vi "Execute Sequence.vi"(4 "Sequence Progress":refnum<vi>, 6 "Pulse Sequence Type":T1, 7 "Sum?":bool=TRUE, 8 "error in (no error)":errorcluster, 9 "file path (use dialog)":path, 10 "Save File":bool, 11 "class objects in":T2) -> (0 "error out":errorcluster, 1 "Stop?":bool, 2 "CMD STR Array":string[](array[string]), 3 "class objects out":T2)   [LabVIEW 2011]
uses:
  Controls/Class Objects.ctl
  Modules/File/Configuration/Configuration.lvclass
  Modules/Hardware/Power Supply/Power Supply.lvclass
  Modules/Hardware/NMR/NMR.lvclass
  Modules/File/TDMS/TDMS.lvclass
  Controls/NMR Pulse Sequence Type.ctl
  Controls/User Interface Action.ctl
  Controls/TDMS File Handling.ctl
  Functional Globals/Pulse Parameters.ctl
  <vilib>/Utility/file.llb/Write To Spreadsheet File (I64).vi
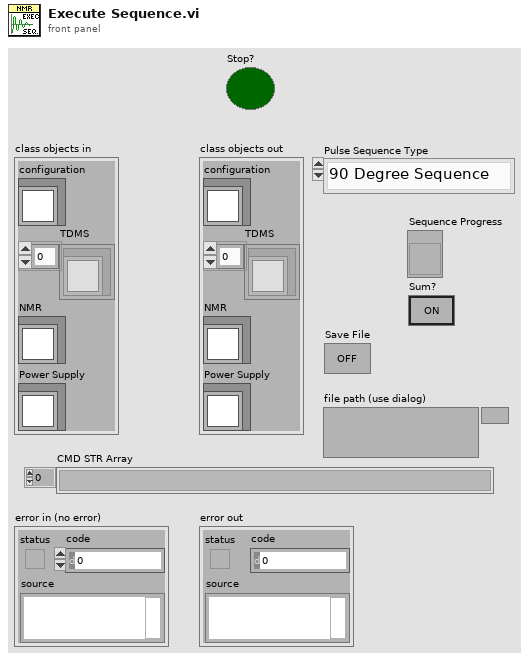
[diagram p1: front panel]
types:
  T1 = typedef "NMR Pulse Sequence Type.ctl" = enum16{"90 Degree Sequence", "CPMG Pulse Sequence", "T1 Pulse Sequence"}
  T2 = typedef "Class Objects.ctl" = cluster{"configuration":refnum<class "Configuration.lvclass">, "TDMS":refnum<class "TDMS.lvclass">[], "Power Supply":refnum<class "Power Supply.lvclass">, "NMR":refnum<class "NMR.lvclass">}
  T3 = typedef "User Interface Action.ctl" = enum16{"Initialize", "Update Real Channel", "Update Imag Channel", "Update Re/Im channel @ Hardware Ctrl", "Pulse Sequence", "Visibility Front Panel Controls", "Report Custom Errors", "Set Pulse Sequence Type", "Update Pulse Timings", "Update Transfer Time", "Update Status Bar", "Set Sequence Progress", "Set 90 Degree Pulse Sequence Params", "Set CMPG Pulse Sequence Parms", "Set T1 Pulse Sequence Params", "Stop"}
  T4 = typedef "TDMS File Handling.ctl" = enum16{"Add TDMS File", "Get Active TDMS File", "Set Active TDMS File", "Set Active TDMS File Index"}
  T5 = typedef "Pulse Parameters.ctl" = enum16{"Initialize", "Set T1 Pulse Settings", "Set 90 Degree Pulse Settings", "Set CPMG Pulse Settings", "Get T1 Settings", "Get CPMG Settings", "Get 90 Degree Settings"}
  T6 = typedef "90D_Delay Settings.ctl" = cluster{"Delay d1":dbl, "Delay d2":dbl, "d1 Unit":u8, "d2 Unit":u8}
  T7 = typedef "90D_Preliminary Settings.ctl" = cluster{"Nº of Scans (ns)":u16, "Pulse Frequency":dbl}
  T8 = typedef "90D_Pulse Settings.ctl" = cluster{"Duration Signal P1":dbl, "Power Level":u16, "Phase":u16, "P1 Units":u8}
  T9 = typedef "Acquisition Settings.ctl" = cluster{"Number Samples":u16, "Time Between Points":dbl, "Unit":u8}
  T10 = cluster{"Delay Settings":T6, "Preliminary Settings":T7, "Pulse Settings":T8, "Acquisition Settings":T9}
  T11 = cluster{"D1 Real Time":ext, "D2 Real Time":ext, "P1 Real Time":ext, "AQS Real Time":ext}
  T12 = typedef "CPMG_Delay Settings.ctl" = cluster{"Delay d1":dbl, "Delay d2":dbl, "d1 Unit":u8, "d2 Unit":u8, "Delay d3":dbl, "d3 Unit":u8, "Delay d4":dbl, "d4 Unit":u8}
  T13 = typedef "CPMG_Preliminary Settings.ctl" = cluster{"Nº of Scans (ns)":u16, "Pulse Frequency":dbl, "Nº of Echoes (ne)":u16}
  T14 = typedef "CPMG_Pulse Settings.ctl" = cluster{"Duration Signal P1":dbl, "Power Level P1":u16, "Phase P1":u16, "P1 Unit":u8, "Duration Signal P2":dbl, "Power Level P2":u16, "Phase P2":u16, "P2 Unit":u8}
  T15 = cluster{"Acquisition Settings":T9, "Delay Settings":T12, "Preliminary Settings":T13, "Pulse Settings":T14}
  T16 = cluster{"Real Time d4":ext, "Real Time d3":ext, "Real Time P2":ext, "Real Time d2":ext, "Real Time P1":ext, "Real Time d1":ext, "Real Time AQS":ext}
  T17 = typedef "T1_Preliminary Settings.ctl" = cluster{"Nº of Scans (ns)":u16, "Pulse Frequency":dbl, "Nº of Vd":u16}
  T18 = typedef "T1_Pulse Settings.ctl" = cluster{"Duration Signal P2":dbl, "Power Level P2":u16, "Phase P2":u16, "P2 Unit":u8, "Duration Signal P1":dbl, "Power Level P1":u16, "Phase P1":u16, "P1 Unit":u8}
  T19 = typedef "T1_Delay Settings.ctl" = cluster{"Delay d1":dbl, "Delay d2":dbl, "d1 Unit":u8, "d2 Unit":u8, "Delay d30":dbl, "d30 Unit":u8, "Vd Unit":u8, "Vd Values":string}
  T20 = cluster{"Preliminary Settings":T17, "Pulse Settings":T18, "Acquisition Settings":T9, "Delay Settings":T19}
  T21 = cluster{"Real Time P1":ext, "Real Time P2":ext, "Real Time d1":ext, "Real Time d2":ext, "Real Time d30":ext, "Real Time AQS":ext}
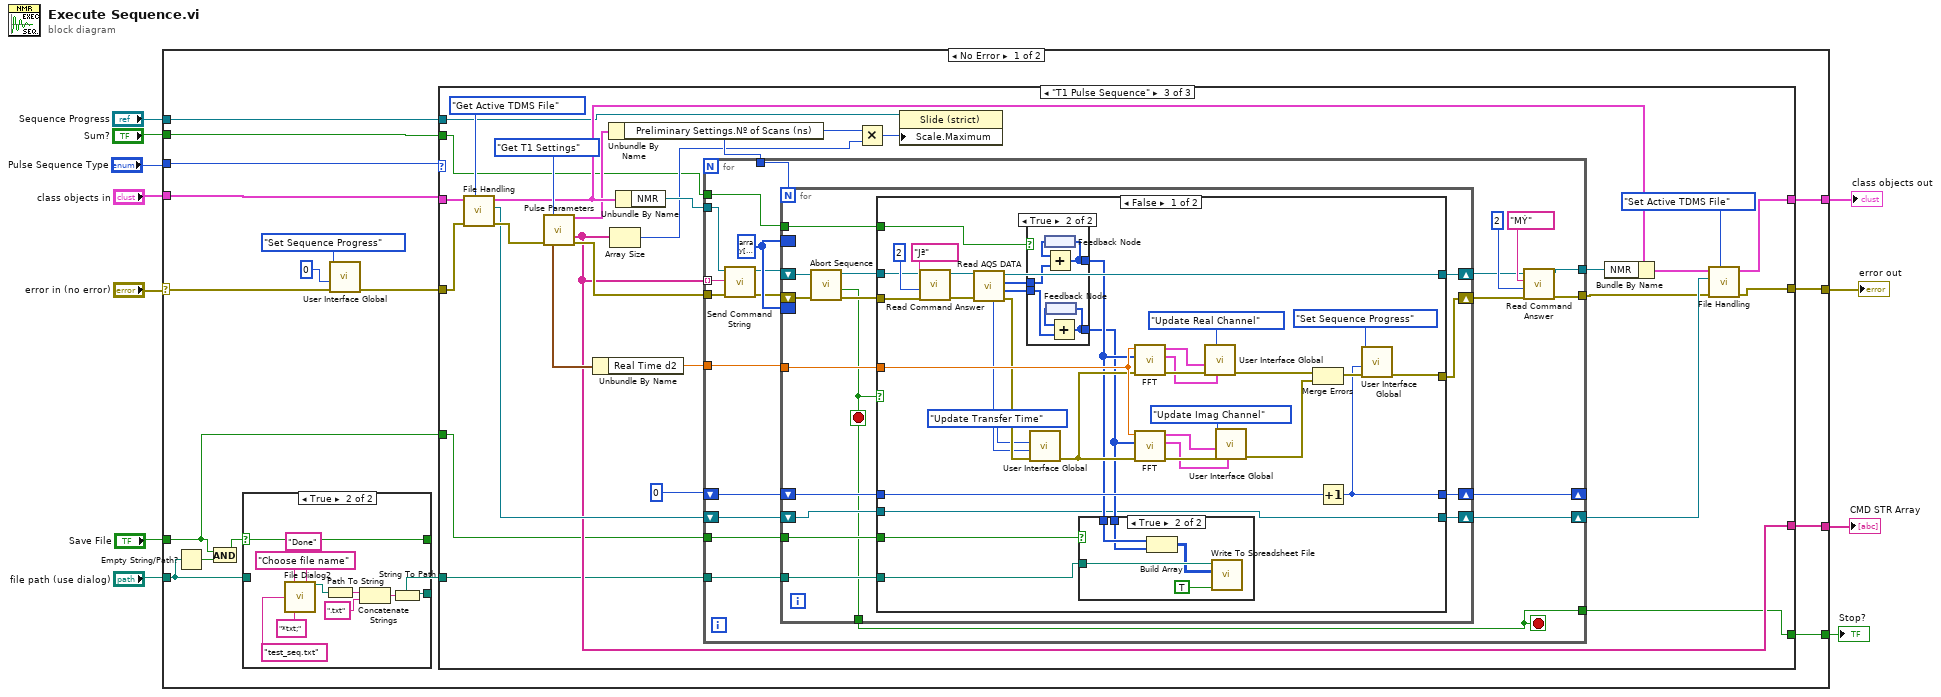
[diagram p0: block diagram]
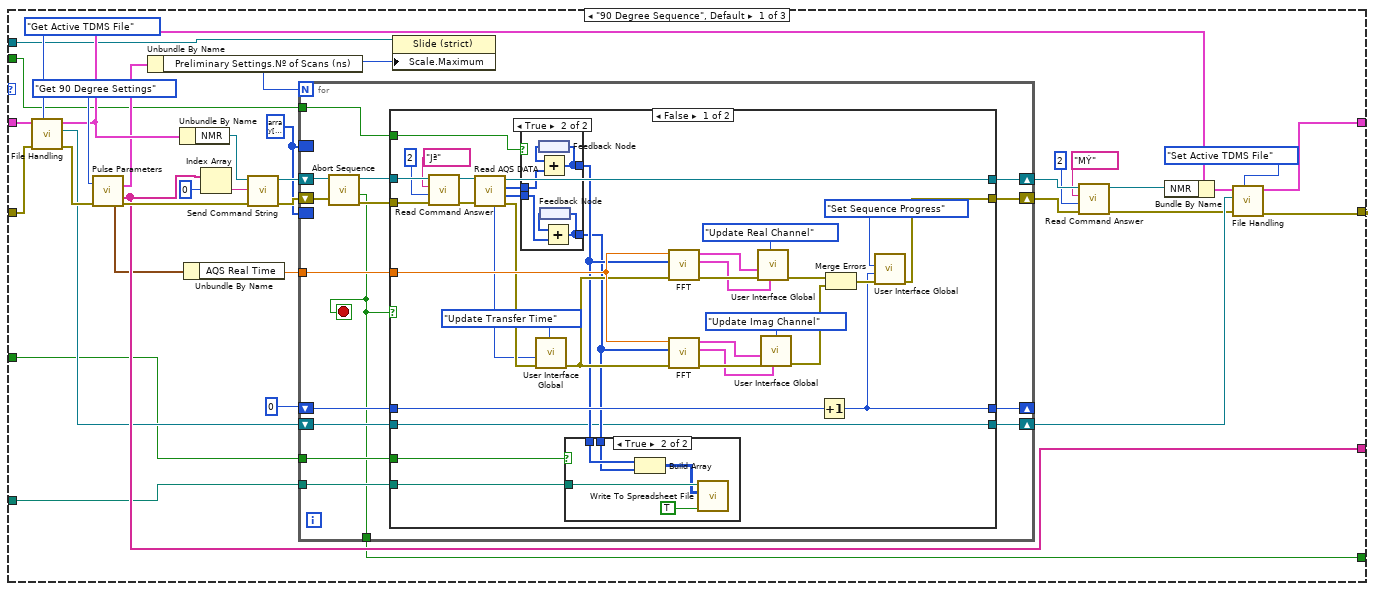
[diagram p3: hidden frame]
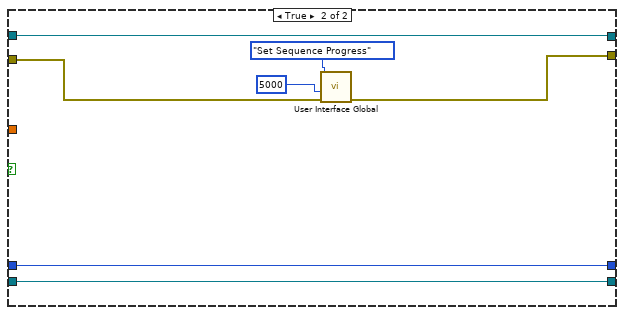
[diagram p6: hidden frame]
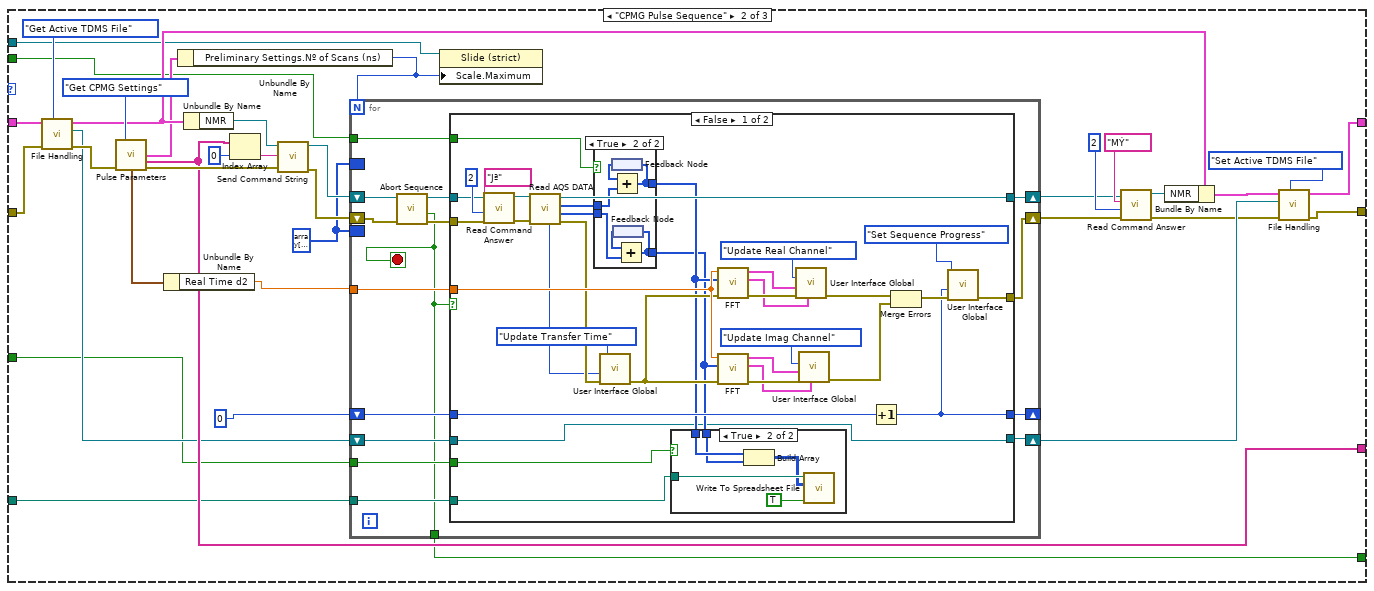
[diagram p7: hidden frame]
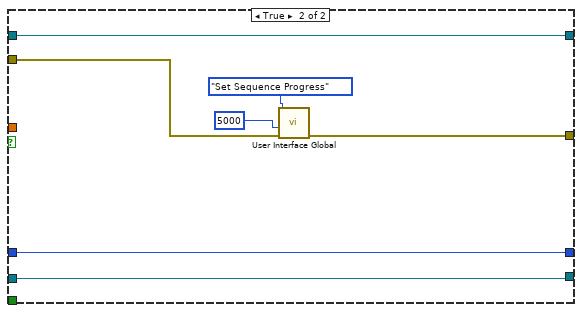
[diagram p10: hidden frame]
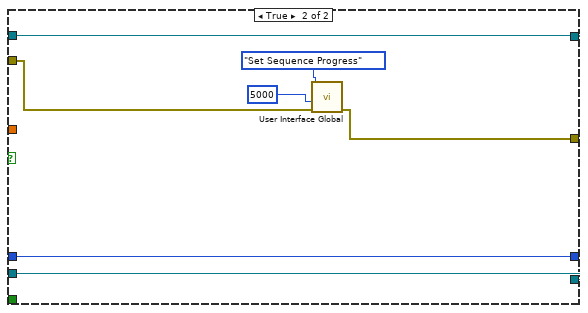
[diagram p13: hidden frame]
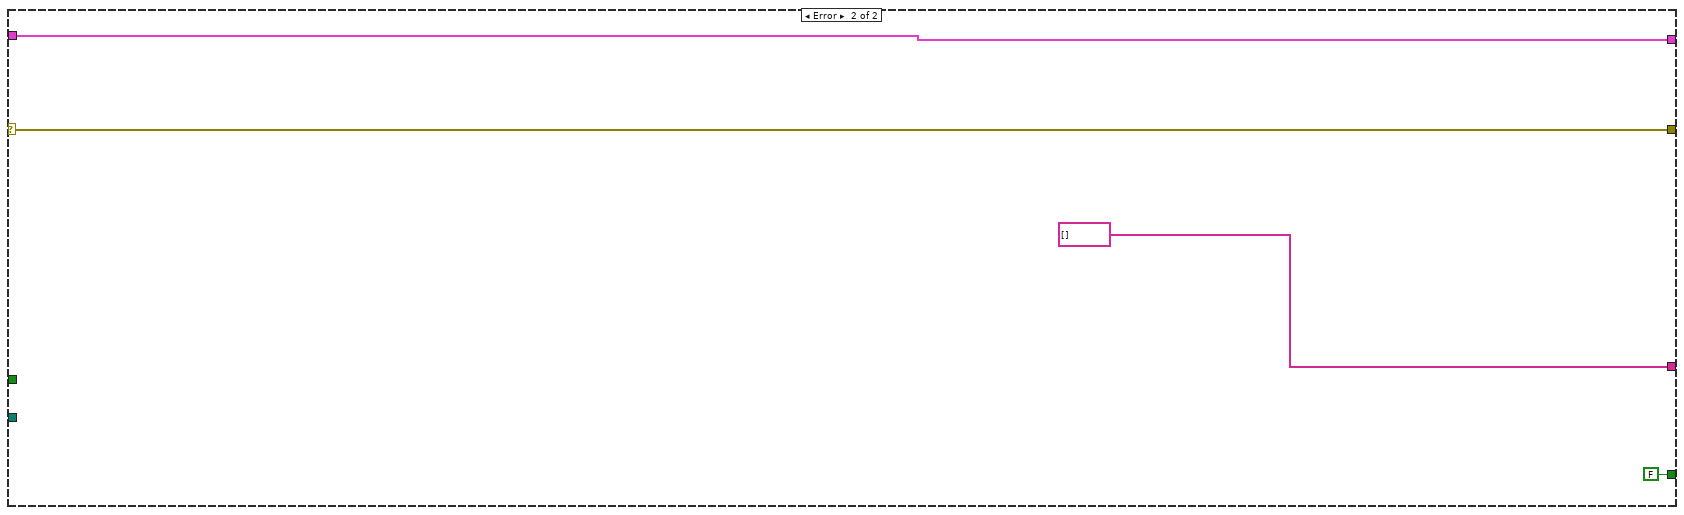
[diagram p14: hidden frame]
diagram:
  n1 = case shown="No Error" "error in (no error)" {
    selector: "error in (no error)" -> [w22 w376]
    tunnel: [w28 string[] [] ("CMD STR Array")] -> w11
    tunnel: [w27 w377] -> w10
    tunnel: "class objects in" -> [w26 w377]
    tunnel: [w25 w376] -> w8
    tunnel: "Pulse Sequence Type" -> [w24 _]
    tunnel: "Sequence Progress" -> [w19 _]
    tunnel: "file path (use dialog)" -> [w15 _]
    tunnel: "Save File" -> [w12 _]
    tunnel: "Sum?" -> [w18 _]
    tunnel: [w17 FALSE ("Stop?")] -> w1
    frame No Error {
      n2 = Empty String/Path?(string/path=w15) -> (empty?=w14:bool)
      n3 = And(x=w12, y=w14) -> (x .and. y?=w13:bool)
      n4 = case shown="True" w13 {
        selector: w13 -> [w30 w40]
        tunnel: [w29 w32] -> w16
        tunnel: [w30 w40] -> _
        tunnel: w15 -> [w29 _]
        frame False {
        }
        frame True {
          n5 = call "File Dialog2"("prompt"="Choose file name", "button label"="Done", "default name"="test_seq.txt" ("button label"), "pattern (all files)"="*txt;" ("pattern")) -> ("selected path"=w31:path)  [unwired: 8 in, 3 out]
          n6 = Path To String(path=w31) -> (string=w35:string)
          n7 = Concatenate Strings(w35, ".txt" ("name or relative path")) -> (w33:string)
          n8 = String To Path(string=w33) -> (path=w32:path)
        }
      }
      n9 = call "User Interface Global.vi"("error in"=w22, "data1"=u8 0 ("Sequence Progress"), "action"=User_Interface_Action."Set Sequence Progress") -> ("error out"=w21:errorcluster)  [unwired: 8 in]
      n10 = case shown="\"T1 Pulse Sequence\"" w24 {
        tunnel: [w72 w178 w261] -> w28
        tunnel: [w57 w164 w268] -> w27
        tunnel: w26 -> [w66 w173 w277]
        tunnel: w21 -> [w63 w170 w274]
        tunnel: [w46 w152 w257] -> w25
        tunnel: w19 -> [w50 w154 w263]
        tunnel: w16 -> [w49 w150 w253]
        tunnel: w12 -> [w48 w149 w255]
        tunnel: w18 -> [w42 w148 w256]
        tunnel: [w41 w147 w254] -> w17
        frame "90 Degree Sequence", Default {
          w43 = i32[] array[9001 elements]
          n11 = call "File Handling.vi"("TDMS File Handling"=TDMS_File_Handling."Get Active TDMS File", "error in"=w63, "objects IN"=w66) -> ("error out"=w62:errorcluster, "TDMS File"=w61:refnum<class "TDMS.lvclass">, "objects OUT"=w65:T2)  [unwired: 6 in]
          n12 = call "Pulse Parameters.vi"("action"=Pulse_Parameters."Get 90 Degree Settings", "error in"=w62) -> ("90 Degree Pulse settings out"=w56:T10, "CMD STR Array"=w72:string[], "Set Time 90 Degree Pulse"=w68:T11, "error out"=w73:errorcluster)  [unwired: 6 in, 4 out]
          n13 = Unbundle By Name(w56) -> ("Preliminary Settings.Nº of Scans (ns)"=w47:u16)
          n14 = Unbundle By Name(w65) -> ("NMR"=w74:refnum<class "NMR.lvclass">)
          n15 = Unbundle By Name(w68) -> ("AQS Real Time"=w67:ext)
          n16 = Index Array(array=w72, index=0) -> (element=w71:string)
          n17 = call-dynamic "Send Command String.vi"("error in (no error)"=w73, "Command String"=w71, "NMR in"=w74) -> ("error out"=w69:errorcluster, "NMR out"=w70:refnum<class "NMR.lvclass">)  [unwired: 7 in]
          n18 = for {
            N: w47 -> [_]
            shift-right: [w86] -> w55
            shift-left: w70 -> [w84]
            shift-right: [w85] -> w54
            shift-left: w69 -> [w83]
            tunnel: w67 -> [w91]
            shift-right: [w79] -> w59
            shift-left: w61 -> [w80]
            shift-right: [w87] -> _
            shift-left: 0 -> [w88]
            tunnel: w49 -> [w90]
            tunnel: w48 -> [w89]
            border: w43 -> [_]
            border: w43 -> [_]
            tunnel: w42 -> [w78]
            tunnel: [w77] -> w41
            stop <- w77 stop-if-true
            n19 = call "Abort Sequence.vi"("error in"=w83, "NMR in"=w84) -> ("error out"=w81:errorcluster, "Stop?"=w77:bool, "NMR out"=w82:refnum<class "NMR.lvclass">)  [unwired: 7 in]
            n20 = case shown="False" w77 {
              tunnel: w91 -> [w120 _]
              tunnel: w90 -> [w115 _]
              tunnel: w89 -> [w114 _]
              tunnel: w88 -> [w113 w145]
              tunnel: [w112 w145] -> w87
              tunnel: [w107 w146] -> w86
              tunnel: [w106 w142] -> w85
              tunnel: w82 -> [w105 w146]
              tunnel: w81 -> [w104 w143]
              tunnel: w80 -> [w93 w140]
              tunnel: [w93 w140] -> w79
              tunnel: w78 -> [w92 _]
              frame False {
                n21 = call-dynamic "Read Command Answer.vi"("error in (no error)"=w104, "bytes to read"=u32 2 ("Number bytes Read"), "String Seached"="Jª" ("search char"), "NMR in"=w105) -> ("error out"=w119:errorcluster, "NMR out"=w118:refnum<class "NMR.lvclass">)  [unwired: 5 in, 1 out]
                n22 = call-dynamic "Read AQS DATA.vi"("error in (no error)"=w119, "NMR in"=w118) -> ("error out"=w111:errorcluster, "Imag Data"=w95:i32[], "Real Data"=w97:i32[], "NMR out"=w107:refnum<class "NMR.lvclass">, "Transfer time"=w108:u32)  [unwired: 5 in]
                n23 = case shown="True" w92 {
                  tunnel: w97 -> [w128 w133]
                  tunnel: [w128 w132] -> w96
                  tunnel: w95 -> [w127 w130]
                  tunnel: [w127 w129] -> w94
                  frame False {
                  }
                  frame True {
                    n24 = feedback #1() -> (w134:i32[])
                    n25 = Add(x=w134, y=w133) -> (x+y=w132:i32[])
                    n26 = feedback-in #1(w132) -> ()
                    n27 = feedback #2() -> (w131:i32[])
                    n28 = Add(x=w131, y=w130) -> (x+y=w129:i32[])
                    n29 = feedback-in #2(w129) -> ()
                  }
                }
                n30 = call "User Interface Global.vi"("error in"=w111, "data1"=w108, "action"=User_Interface_Action."Update Transfer Time") -> ("error out"=w110:errorcluster)  [unwired: 8 in]
                n31 = case shown="True" w114 {
                  tunnel: w96 -> [_ w137]
                  tunnel: w94 -> [_ w136]
                  tunnel: w115 -> [_ w138]
                  frame False {
                  }
                  frame True {
                    n32 = Build Array(w137, w136) -> (w135:i32[][])
                    n33 = call-poly <vilib>:"Write To Spreadsheet File.vi"("append to file? (new file:F)"=TRUE, "2D data"=w135, "file path (dialog if empty)"=w138) -> ()  [unwired: 5 in, 1 out]
                  }
                }
                n34 = call "FFT.vi"("error in (no error)"=w110, "Input Array"=w96, "Delay Sample"=w120) -> ("error out"=w125:errorcluster, "Time Graph"=w103:cluster{"magnitude":dbl[], dbl[]}, "FFT Graph"=w126:cluster{"magnitude":dbl[], dbl[]})  [unwired: 6 in]
                n35 = call "FFT.vi"("error in (no error)"=w110, "Input Array"=w94, "Delay Sample"=w120) -> ("error out"=w122:errorcluster, "Time Graph"=w101:cluster{"magnitude":dbl[], dbl[]}, "FFT Graph"=w121:cluster{"magnitude":dbl[], dbl[]})  [unwired: 6 in]
                n36 = call "User Interface Global.vi"("data2"=w103, "error in"=w125, "data1"=w126, "action"=User_Interface_Action."Update Real Channel") -> ("error out"=w102:errorcluster)  [unwired: 7 in]
                n37 = call "User Interface Global.vi"("data2"=w101, "error in"=w122, "data1"=w121, "action"=User_Interface_Action."Update Imag Channel") -> ("error out"=w100:errorcluster)  [unwired: 7 in]
                n38 = Increment(x=w113) -> (x+1=w112:i32)
                n39 = Merge Errors(w102, w100) -> (w116:errorcluster)
                n40 = call "User Interface Global.vi"("error in"=w116, "data1"=w112, "action"=User_Interface_Action."Set Sequence Progress") -> ("error out"=w106:errorcluster)  [unwired: 8 in]
              }
              frame True {
                n41 = call "User Interface Global.vi"("error in"=w143, "data1"=5000, "action"=User_Interface_Action."Set Sequence Progress") -> ("error out"=w142:errorcluster)  [unwired: 8 in]
              }
            }
          }
          n42 = property class="Slide (strict)"(reference=w50, "Scale.Maximum"=w47) -> ()  [unwired: 1 in, 2 out]
          n43 = call-dynamic "Read Command Answer.vi"("error in (no error)"=w54, "bytes to read"=u32 2 ("Number bytes Read"), "String Seached"="MÝ" ("search char"), "NMR in"=w55) -> ("error out"=w53:errorcluster, "NMR out"=w52:refnum<class "NMR.lvclass">)  [unwired: 5 in, 1 out]
          n44 = Bundle By Name(cluster=w65, "NMR"=w52) -> (w58:T2)
          n45 = call "File Handling.vi"("TDMS File Handling"=TDMS_File_Handling."Set Active TDMS File", "error in"=w53, "TDMS File"=w59, "objects IN"=w58) -> ("error out"=w46:errorcluster, "objects OUT"=w57:T2)  [unwired: 5 in, 1 out]
        }
        frame "CPMG Pulse Sequence" {
          w151 = i32[] array[9001 elements]
          n46 = call "File Handling.vi"("TDMS File Handling"=TDMS_File_Handling."Get Active TDMS File", "error in"=w170, "objects IN"=w173) -> ("error out"=w169:errorcluster, "TDMS File"=w168:refnum<class "TDMS.lvclass">, "objects OUT"=w172:T2)  [unwired: 6 in]
          n47 = call "Pulse Parameters.vi"("action"=Pulse_Parameters."Get CPMG Settings", "error in"=w169) -> ("CPMG pulse settings Out"=w163:T15, "CMD STR Array"=w178:string[], "CPMG Set Times"=w162:T16, "error out"=w179:errorcluster)  [unwired: 6 in, 4 out]
          n48 = Unbundle By Name(w162) -> ("Real Time d2"=w174:ext)
          n49 = Unbundle By Name(w163) -> ("Preliminary Settings.Nº of Scans (ns)"=w153:u16)
          n50 = Unbundle By Name(w172) -> ("NMR"=w180:refnum<class "NMR.lvclass">)
          n51 = Index Array(array=w178, index=0) -> (element=w177:string)
          n52 = call-dynamic "Send Command String.vi"("error in (no error)"=w179, "Command String"=w177, "NMR in"=w180) -> ("error out"=w175:errorcluster, "NMR out"=w176:refnum<class "NMR.lvclass">)  [unwired: 7 in]
          n53 = for {
            N: w153 -> [_]
            shift-right: [w197] -> w159
            shift-left: w176 -> [w192]
            shift-right: [w195] -> w158
            shift-left: w175 -> [w191]
            tunnel: w174 -> [w196]
            shift-right: [w185] -> w166
            shift-left: w168 -> [w186]
            shift-right: [w193] -> _
            shift-left: 0 -> [w194]
            border: w151 -> [_]
            border: w151 -> [_]
            tunnel: w150 -> [w188]
            tunnel: w149 -> [w187]
            tunnel: w148 -> [w184]
            tunnel: [w183] -> w147
            stop <- w183 stop-if-true
            n54 = call "Abort Sequence.vi"("error in"=w191, "NMR in"=w192) -> ("error out"=w190:errorcluster, "Stop?"=w183:bool, "NMR out"=w189:refnum<class "NMR.lvclass">)  [unwired: 7 in]
            n55 = case shown="False" w183 {
              tunnel: [w226 w252] -> w197
              tunnel: w196 -> [w225 _]
              tunnel: [w220 w248] -> w195
              tunnel: w194 -> [w219 w247]
              tunnel: [w218 w247] -> w193
              tunnel: w190 -> [w207 w249]
              tunnel: w189 -> [w206 w252]
              tunnel: w188 -> [w201 _]
              tunnel: w187 -> [w200 _]
              tunnel: [w199 w246] -> w185
              tunnel: w186 -> [w199 w246]
              tunnel: w184 -> [w198 _]
              frame False {
                n56 = call-dynamic "Read Command Answer.vi"("error in (no error)"=w207, "bytes to read"=u32 2 ("Number bytes Read"), "String Seached"="Jª" ("search char"), "NMR in"=w206) -> ("error out"=w224:errorcluster, "NMR out"=w223:refnum<class "NMR.lvclass">)  [unwired: 5 in, 1 out]
                n57 = call-dynamic "Read AQS DATA.vi"("error in (no error)"=w224, "NMR in"=w223) -> ("error out"=w217:errorcluster, "Imag Data"=w204:i32[], "Real Data"=w205:i32[], "NMR out"=w226:refnum<class "NMR.lvclass">, "Transfer time"=w215:u32)  [unwired: 5 in]
                n58 = case shown="True" w198 {
                  tunnel: w205 -> [w239 w244]
                  tunnel: [w239 w243] -> w203
                  tunnel: w204 -> [w238 w241]
                  tunnel: [w238 w240] -> w202
                  frame False {
                  }
                  frame True {
                    n59 = feedback #3() -> (w245:i32[])
                    n60 = Add(x=w245, y=w244) -> (x+y=w243:i32[])
                    n61 = feedback-in #3(w243) -> ()
                    n62 = feedback #4() -> (w242:i32[])
                    n63 = Add(x=w242, y=w241) -> (x+y=w240:i32[])
                    n64 = feedback-in #4(w240) -> ()
                  }
                }
                n65 = call "User Interface Global.vi"("error in"=w217, "data1"=w215, "action"=User_Interface_Action."Update Transfer Time") -> ("error out"=w216:errorcluster)  [unwired: 8 in]
                n66 = case shown="True" w200 {
                  tunnel: w203 -> [_ w235]
                  tunnel: w202 -> [_ w234]
                  tunnel: w201 -> [_ w236]
                  frame False {
                  }
                  frame True {
                    n67 = Build Array(w235, w234) -> (w233:i32[][])
                    n68 = call-poly <vilib>:"Write To Spreadsheet File.vi"("append to file? (new file:F)"=TRUE, "2D data"=w233, "file path (dialog if empty)"=w236) -> ()  [unwired: 5 in, 1 out]
                  }
                }
                n69 = call "FFT.vi"("error in (no error)"=w216, "Input Array"=w203, "Delay Sample"=w225) -> ("error out"=w231:errorcluster, "Time Graph"=w213:cluster{"magnitude":dbl[], dbl[]}, "FFT Graph"=w232:cluster{"magnitude":dbl[], dbl[]})  [unwired: 6 in]
                n70 = call "FFT.vi"("error in (no error)"=w216, "Input Array"=w202, "Delay Sample"=w225) -> ("error out"=w228:errorcluster, "Time Graph"=w211:cluster{"magnitude":dbl[], dbl[]}, "FFT Graph"=w227:cluster{"magnitude":dbl[], dbl[]})  [unwired: 6 in]
                n71 = call "User Interface Global.vi"("data2"=w213, "error in"=w231, "data1"=w232, "action"=User_Interface_Action."Update Real Channel") -> ("error out"=w212:errorcluster)  [unwired: 7 in]
                n72 = call "User Interface Global.vi"("data2"=w211, "error in"=w228, "data1"=w227, "action"=User_Interface_Action."Update Imag Channel") -> ("error out"=w210:errorcluster)  [unwired: 7 in]
                n73 = Increment(x=w219) -> (x+1=w218:i32)
                n74 = Merge Errors(w212, w210) -> (w221:errorcluster)
                n75 = call "User Interface Global.vi"("error in"=w221, "data1"=w218, "action"=User_Interface_Action."Set Sequence Progress") -> ("error out"=w220:errorcluster)  [unwired: 8 in]
              }
              frame True {
                n76 = call "User Interface Global.vi"("error in"=w249, "data1"=5000, "action"=User_Interface_Action."Set Sequence Progress") -> ("error out"=w248:errorcluster)  [unwired: 8 in]
              }
            }
          }
          n77 = property class="Slide (strict)"(reference=w154, "Scale.Maximum"=w153) -> ()  [unwired: 1 in, 2 out]
          n78 = call-dynamic "Read Command Answer.vi"("error in (no error)"=w158, "bytes to read"=u32 2 ("Number bytes Read"), "String Seached"="MÝ" ("search char"), "NMR in"=w159) -> ("error out"=w157:errorcluster, "NMR out"=w156:refnum<class "NMR.lvclass">)  [unwired: 5 in, 1 out]
          n79 = Bundle By Name(cluster=w172, "NMR"=w156) -> (w165:T2)
          n80 = call "File Handling.vi"("TDMS File Handling"=TDMS_File_Handling."Set Active TDMS File", "error in"=w157, "TDMS File"=w166, "objects IN"=w165) -> ("error out"=w152:errorcluster, "objects OUT"=w164:T2)  [unwired: 5 in, 1 out]
        }
        frame "T1 Pulse Sequence" {
          n81 = call "File Handling.vi"("TDMS File Handling"=TDMS_File_Handling."Get Active TDMS File", "error in"=w274, "objects IN"=w277) -> ("error out"=w273:errorcluster, "TDMS File"=w272:refnum<class "TDMS.lvclass">, "objects OUT"=w276:T2)  [unwired: 6 in]
          n82 = call "Pulse Parameters.vi"("action"=Pulse_Parameters."Get T1 Settings", "error in"=w273) -> ("T1 Pulse settings Out"=w266:T20, "CMD STR Array"=w261:string[], "T1 set times"=w267:T21, "error out"=w279:errorcluster)  [unwired: 6 in, 4 out]
          n83 = Unbundle By Name(w267) -> ("Real Time d2"=w278:ext)
          n84 = Unbundle By Name(w266) -> ("Preliminary Settings.Nº of Scans (ns)"=w262:u16)
          n85 = Array Size(array=w261) -> (size(s)=w260:i32)
          n86 = Unbundle By Name(w276) -> ("NMR"=w280:refnum<class "NMR.lvclass">)
          n87 = for {
            tunnel: w280 -> [w303]
            tunnel: w279 -> [w302]
            tunnel: w261 -> [w301] mode=indexing
            tunnel: w278 -> [w300]
            shift-right: [w298] -> w270
            shift-left: w272 -> [w299]
            tunnel: w262 -> [w291]
            tunnel: [w293] -> w265
            tunnel: [w292] -> w264
            shift-right: [w290] -> _
            shift-left: 0 -> [w289]
            tunnel: w256 -> [w288]
            tunnel: w253 -> [w287]
            tunnel: w255 -> [w286]
            tunnel: [w282] -> w254
            stop <- w282 stop-if-true
            w285 = i32[] array[9001 elements]
            n88 = call-dynamic "Send Command String.vi"("error in (no error)"=w302, "Command String"=w301, "NMR in"=w303) -> ("error out"=w283:errorcluster, "NMR out"=w284:refnum<class "NMR.lvclass">)  [unwired: 7 in]
            n89 = for {
              N: w291 -> [_]
              shift-right: [w318] -> w295
              shift-left: w284 -> [w308]
              shift-right: [w316] -> w294
              shift-left: w283 -> [w307]
              tunnel: w300 -> [w317]
              shift-right: [w309] -> w298
              shift-left: w299 -> [w310]
              shift-right: [w314] -> w290
              shift-left: w289 -> [w315]
              tunnel: w288 -> [w313]
              tunnel: w287 -> [w312]
              tunnel: w286 -> [w311]
              border: w285 -> [_]
              border: w285 -> [_]
              tunnel: [w304] -> w282
              stop <- w304 stop-if-true
              n90 = call "Abort Sequence.vi"("error in"=w307, "NMR in"=w308) -> ("error out"=w306:errorcluster, "Stop?"=w304:bool, "NMR out"=w305:refnum<class "NMR.lvclass">)  [unwired: 7 in]
              n91 = case shown="False" w304 {
                tunnel: [w347 w371] -> w318
                tunnel: w317 -> [w346 _]
                tunnel: [w339 w369] -> w316
                tunnel: w315 -> [w338 w368]
                tunnel: [w337 w368] -> w314
                tunnel: w305 -> [w328 w371]
                tunnel: w306 -> [w327 w370]
                tunnel: w313 -> [w324 _]
                tunnel: w312 -> [w321 _]
                tunnel: w311 -> [w320 _]
                tunnel: [w319 w367] -> w309
                tunnel: w310 -> [w319 w367]
                frame False {
                  n92 = call-dynamic "Read Command Answer.vi"("error in (no error)"=w327, "bytes to read"=u32 2 ("Number bytes Read"), "String Seached"="Jª" ("search char"), "NMR in"=w328) -> ("error out"=w343:errorcluster, "NMR out"=w342:refnum<class "NMR.lvclass">)  [unwired: 5 in, 1 out]
                  n93 = call-dynamic "Read AQS DATA.vi"("error in (no error)"=w343, "NMR in"=w342) -> ("error out"=w336:errorcluster, "Imag Data"=w325:i32[], "Real Data"=w326:i32[], "NMR out"=w347:refnum<class "NMR.lvclass">, "Transfer time"=w334:u32)  [unwired: 5 in]
                  n94 = case shown="True" w324 {
                    tunnel: w326 -> [w360 w365]
                    tunnel: [w360 w364] -> w323
                    tunnel: w325 -> [w359 w362]
                    tunnel: [w359 w361] -> w322
                    frame False {
                    }
                    frame True {
                      n95 = feedback #5() -> (w366:i32[])
                      n96 = Add(x=w366, y=w365) -> (x+y=w364:i32[])
                      n97 = feedback-in #5(w364) -> ()
                      n98 = feedback #6() -> (w363:i32[])
                      n99 = Add(x=w363, y=w362) -> (x+y=w361:i32[])
                      n100 = feedback-in #6(w361) -> ()
                    }
                  }
                  n101 = call "User Interface Global.vi"("error in"=w336, "data1"=w334, "action"=User_Interface_Action."Update Transfer Time") -> ("error out"=w335:errorcluster)  [unwired: 8 in]
                  n102 = case shown="True" w320 {
                    tunnel: w323 -> [_ w356]
                    tunnel: w322 -> [_ w355]
                    tunnel: w321 -> [_ w357]
                    frame False {
                    }
                    frame True {
                      n103 = Build Array(w356, w355) -> (w354:i32[][])
                      n104 = call-poly <vilib>:"Write To Spreadsheet File.vi"("append to file? (new file:F)"=TRUE, "2D data"=w354, "file path (dialog if empty)"=w357) -> ()  [unwired: 5 in, 1 out]
                    }
                  }
                  n105 = call "FFT.vi"("error in (no error)"=w335, "Input Array"=w323, "Delay Sample"=w346) -> ("error out"=w352:errorcluster, "Time Graph"=w331:cluster{"magnitude":dbl[], dbl[]}, "FFT Graph"=w353:cluster{"magnitude":dbl[], dbl[]})  [unwired: 6 in]
                  n106 = call "FFT.vi"("error in (no error)"=w335, "Input Array"=w322, "Delay Sample"=w346) -> ("error out"=w349:errorcluster, "Time Graph"=w332:cluster{"magnitude":dbl[], dbl[]}, "FFT Graph"=w348:cluster{"magnitude":dbl[], dbl[]})  [unwired: 6 in]
                  n107 = call "User Interface Global.vi"("data2"=w331, "error in"=w352, "data1"=w353, "action"=User_Interface_Action."Update Real Channel") -> ("error out"=w330:errorcluster)  [unwired: 7 in]
                  n108 = call "User Interface Global.vi"("data2"=w332, "error in"=w349, "data1"=w348, "action"=User_Interface_Action."Update Imag Channel") -> ("error out"=w329:errorcluster)  [unwired: 7 in]
                  n109 = Merge Errors(w330, w329) -> (w340:errorcluster)
                  n110 = Increment(x=w338) -> (x+1=w337:i32)
                  n111 = call "User Interface Global.vi"("error in"=w340, "data1"=w337, "action"=User_Interface_Action."Set Sequence Progress") -> ("error out"=w339:errorcluster)  [unwired: 8 in]
                }
                frame True {
                  n112 = call "User Interface Global.vi"("error in"=w370, "data1"=5000, "action"=User_Interface_Action."Set Sequence Progress") -> ("error out"=w369:errorcluster)  [unwired: 8 in]
                }
              }
            }
            n113 = call-dynamic "Read Command Answer.vi"("error in (no error)"=w294, "bytes to read"=u32 2 ("Number bytes Read"), "String Seached"="MÝ" ("search char"), "NMR in"=w295) -> ("error out"=w292:errorcluster, "NMR out"=w293:refnum<class "NMR.lvclass">)  [unwired: 5 in, 1 out]
          }
          n114 = Multiply(x=w262, y=w260) -> (x*y=w258:i32)
          n115 = property class="Slide (strict)"(reference=w263, "Scale.Maximum"=w258) -> ()  [unwired: 1 in, 2 out]
          n116 = Bundle By Name(cluster=w276, "NMR"=w265) -> (w269:T2)
          n117 = call "File Handling.vi"("TDMS File Handling"=TDMS_File_Handling."Set Active TDMS File", "error in"=w264, "TDMS File"=w270, "objects IN"=w269) -> ("error out"=w257:errorcluster, "objects OUT"=w268:T2)  [unwired: 5 in, 1 out]
        }
      }
    }
    frame Error {
    }
  }
  "CMD STR Array" <- w11
  "class objects out" <- w10
  "error out" <- w8
  "Stop?" <- w1
